vi "GetDevicesInfo.vi"(8 "error in (no error)":errorcluster) -> (0 "error out":errorcluster, 1 "mouse info":T3(array[cluster]), 2 "key info":T2(array[cluster]), 3 "joystick info":T1(array[cluster]))   [LabVIEW 2021, in "InputDevice.lvlib" / "InputDevice.lvclass"]
uses:
  InputDevice.lvclass
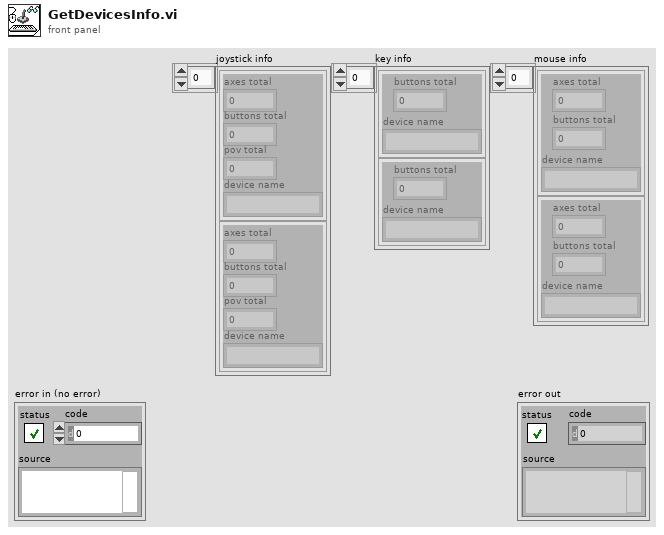
[diagram p1: front panel]
types:
  T1 = cluster{"axes total":u32, "buttons total":u32, "pov total":u32, "device name":string}[]
  T2 = cluster{"buttons total":u32, "device name":string}[]
  T3 = cluster{"axes total":u32, "buttons total":u32, "device name":string}[]
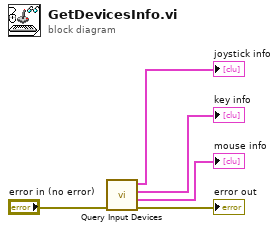
[diagram p0: block diagram]
diagram:
  n1 = call <vilib>:"Query Input Devices.vi"("error in (no error)"="error in (no error)") -> ("error out"=→"error out":errorcluster, "mouse info"=→"mouse info":T3, "key info"=→"key info":T2, "joystick info"=→"joystick info":T1)  [unwired: 7 in]
